vi "Exemple_PropsSI.vi"() -> ()   [LabVIEW 2020]
panel:
  in  "stop":bool
  out "String":string
  in  "Fluids name":i32(listbox)
  in  "Second known var\nvalue":dbl=1.0
  in  "Second known var":string="Q"
  in  "First known var\nvalue":dbl
  in  "First known\nvar":string="P"
  in  "Desired var":string="T"
  out "return value":dbl
  out "error out":errorcluster
  in  "error in (no error)":errorcluster
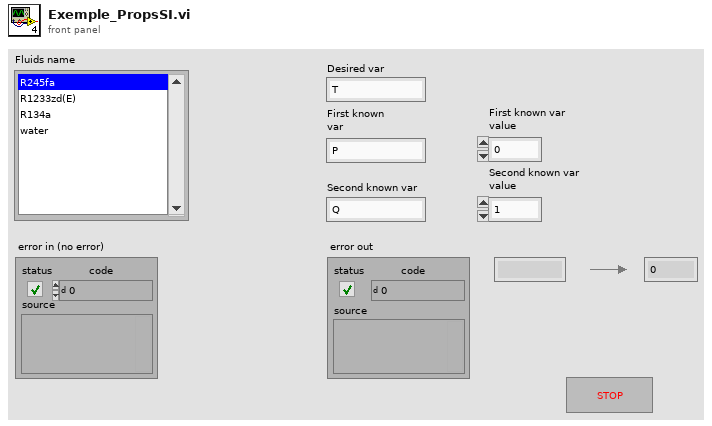
[diagram p1: front panel]
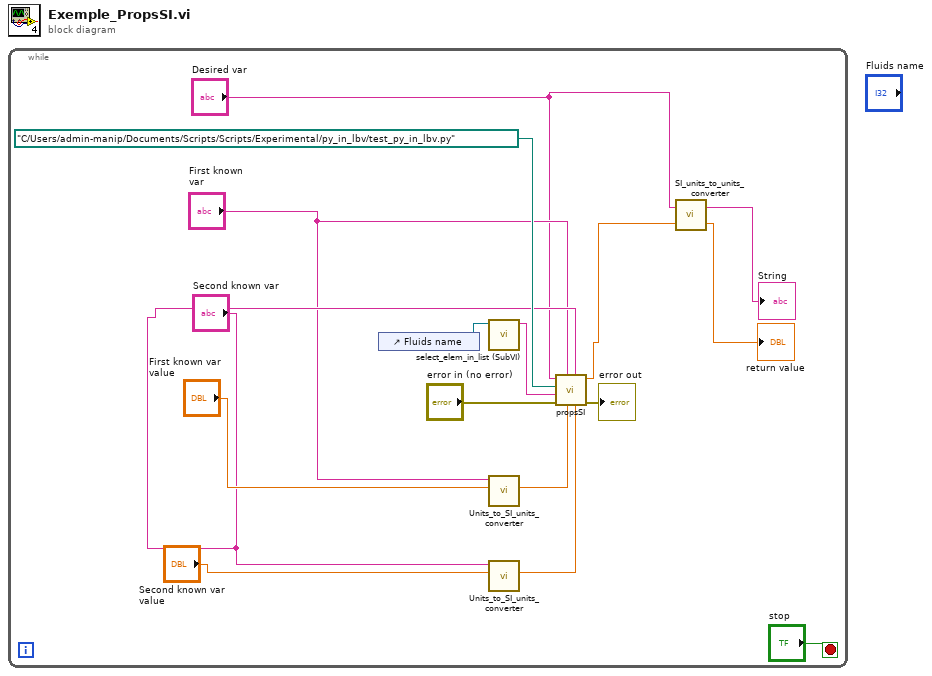
[diagram p0: block diagram]
diagram:
  n1 = while {
    stop <- "stop" stop-if-true
    n2 = control-ref of="Fluids name"() -> (w13:refnum<vi>)
    n3 = call "select_elem_in_list (SubVI).vi"("ListBox in"=w13) -> ("String"=w12:string)  [unwired: 10 in]
    n4 = call "Units_to_SI_units_converter.vi"("var_value in"="First known var\nvalue", "String in"="First known\nvar") -> ("var_value out"=w11:dbl)  [unwired: 8 in, 1 out]
    n5 = call "Units_to_SI_units_converter.vi"("var_value in"="Second known var\nvalue", "String in"="Second known var") -> ("var_value out"=w10:dbl)  [unwired: 8 in, 1 out]
    n6 = call "propsSI.vi"("Second known var value [SI]"=w10, "Second known var"="Second known var", "First known var value [SI]"=w11, "First known\nvar"="First known\nvar", "error in (no error)"="error in (no error)", "Fluid"=w12, "module path"=path "C:/Users/admin-manip/Documents/Scripts/Scripts/Experimental/py_in_lbv/test_py_in_lbv.py", "Desired var in"="Desired var") -> ("error out"=→"error out":errorcluster, "Output [SI]"=w7:dbl)  [unwired: 2 in]
    n7 = call "SI_units_to_units_converter.vi"("var_value in"=w7, "String in"="Desired var") -> ("var_value out"=→"return value":dbl, "String out"=→"String":string)
  }
